vi "Euler Angles To Direction Cosines.vi"(10 "rotation order":T1=10 items=["X-Y-Z", "X-Z-Y", "Y-X-Z", "Y-Z-X", "Z-X-Y", "Z-Y-X", "X-Y-X", "X-Z-X", "Y-X-Y", "Y-Z-Y", "Z-X-Z", "Z-Y-Z"], 11 "Euler Angles":cluster{"phi":dbl, "theta":dbl, "psi":dbl}) -> (0 "error":i32, 3 "Direction Cosines":dbl[][](array[numeric]))   [LabVIEW 2017, in "NI_AALPro.lvlib"]
doc: "Converts Euler angles into a 3-by-3 matrix of direction cosines. The VI accepts both proper and Tait-Bryan angle types."
uses:
  NI_AALPro.lvlib
  Euler Rotation Order.ctl
  <resource>/lvanlys.dll
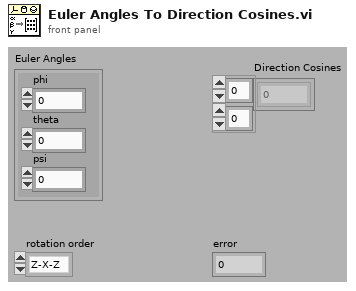
[diagram p1: front panel]
types:
  T1 = typedef "NI_AALPro.lvlib/Euler Rotation Order.ctl" = u16
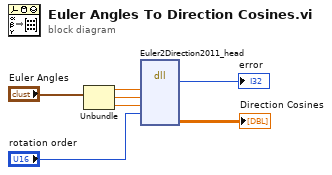
[diagram p0: block diagram]
diagram:
  n1 = Unbundle("Euler Angles") -> ("phi"=w6:dbl, "theta"=w5:dbl, "psi"=w4:dbl)
  n2 = dll-call lib="C:/Program Files (x86)/National Instruments/LabVIEW 2017/resource/lvanlys.*" fn="Euler2Direction2011_head"("phi"=w6, "theta"=w5, "psi"=w4, "rotateOrder"="rotation order") -> ("return type"=→"error":i32, "direction"=→"Direction Cosines":dbl[][])  [unwired: 8 in, 2 out]
